vi "Presets.vi"(4 "RLimit":bool, 6 "LLimit":bool, 8 "TwistAxis":dbl, 9 "Key":bool, 10 "STOP":bool, 11 "100":bool) -> ()   [LabVIEW 2011]
uses:
  Manual-Auto.vi
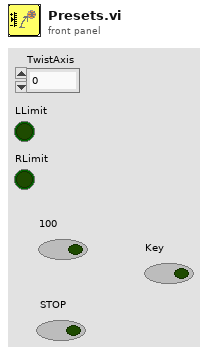
[diagram p1: front panel]
types:
  T1 = typedef "WPI_MotorControlDeviceRef.ctl" = cluster{"DeviceStatus":errorcluster, "Type":enum16{"PWM", "CAN"}, "PWM":cluster{"Digital Module":T2, "PWM Channel":T3, "DeadBand":T4}, "CAN":cluster{"Device Number":u8, "Control Mode":T5, "Semaphore":T6, "Max Vout":dbl}, "Invert":bool, "TransformRef":T7, "InvTransformRef":T7}
  T2 = typedef "FPGA_TypedefDigitalModule.ctl" = enum16{"Digital Module 1", "Digital Module 2"}
  T3 = typedef "FPGA_DIOPWMChannel.ctl" = enum8{"PWM 1", "PWM 2", "PWM 3", "PWM 4", "PWM 5", "PWM 6", "PWM 7", "PWM 8", "PWM 9", "PWM 10", "Invalid"}
  T4 = typedef "WPI_PWMDeadband.ctl" = cluster{"Name":string, "maxPositivePwm":i32, "minPositivePwm":i32, "centerPwm":i32, "maxNegativePwm":i32, "minNegativePwm":i32, "angularRange":u16}
  T5 = typedef "WPI_CANJaguar_ControlMode.ctl" = enum8{"Percent VBus", "Current", "Speed", "Position", "Voltage"}
  T6 = typedef "Semaphore RefNum" = refnum<k1>
  T7 = typedef "WPI_PWMTransform_ConPane.ctl" = refnum<vi>
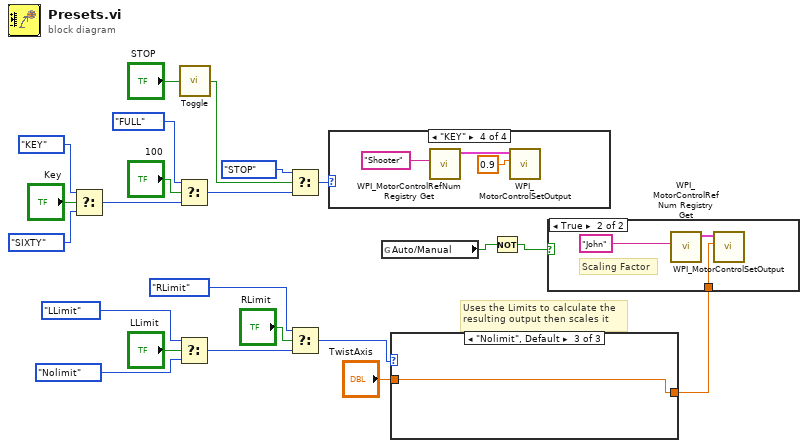
[diagram p0: block diagram]
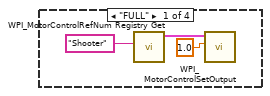
[diagram p3: hidden frame]
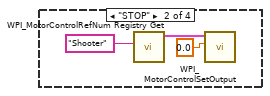
[diagram p4: hidden frame]
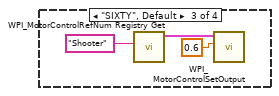
[diagram p5: hidden frame]
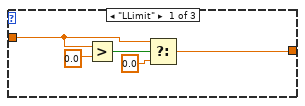
[diagram p6: hidden frame]
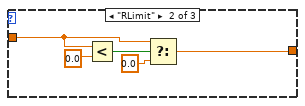
[diagram p7: hidden frame]
diagram:
  # "Uses the Limits to calculate the\nresulting output then scales it"
  n1 = Select(t=enum16{"FULL", "STOP", "SIXTY", "KEY"}."KEY", s="Key", f=enum16{"FULL", "STOP", "SIXTY", "KEY"}."SIXTY") -> (s? t:f=w10:enum16{"FULL", "STOP", "SIXTY", "KEY"})
  n2 = Select(t=enum16{"FULL", "STOP", "SIXTY", "KEY"}."FULL", s="100", f=w10) -> (s? t:f=w13:enum16{"FULL", "STOP", "SIXTY", "KEY"})
  n3 = Select(t=enum16{"LLimit", "RLimit", "Nolimit"}."LLimit", s="LLimit", f=enum16{"LLimit", "RLimit", "Nolimit"}."Nolimit") -> (s? t:f=w20:enum16{"LLimit", "RLimit", "Nolimit"})
  n4 = call "Toggle.vi"("Boolean"="STOP") -> ("Boolean 2"=w3:bool)
  n5 = Select(t=enum16{"FULL", "STOP", "SIXTY", "KEY"}."STOP", s=w3, f=w13) -> (s? t:f=w12:enum16{"FULL", "STOP", "SIXTY", "KEY"})
  n6 = Select(t=enum16{"LLimit", "RLimit", "Nolimit"}."RLimit", s="RLimit", f=w20) -> (s? t:f=w18:enum16{"LLimit", "RLimit", "Nolimit"})
  n7 = case shown="\"KEY\"" w12 {
    frame "FULL" {
      n8 = call <vilib>:"WPI_MotorControlRefNum Registry Get.vi"("refnum name"="Shooter") -> ("MotorControlDevRef"=w23:T1)  [unwired: 9 in, 1 out]
      n9 = call <vilib>:"WPI_MotorControlSetOutput.vi"("Output"=1.0, "MotorControlDevRef"=w23) -> ()  [unwired: 8 in, 2 out]
    }
    frame "STOP" {
      n10 = call <vilib>:"WPI_MotorControlRefNum Registry Get.vi"("refnum name"="Shooter") -> ("MotorControlDevRef"=w28:T1)  [unwired: 9 in, 1 out]
      n11 = call <vilib>:"WPI_MotorControlSetOutput.vi"("Output"=0.0, "MotorControlDevRef"=w28) -> ()  [unwired: 8 in, 2 out]
    }
    frame "SIXTY", Default {
      n12 = call <vilib>:"WPI_MotorControlRefNum Registry Get.vi"("refnum name"="Shooter") -> ("MotorControlDevRef"=w31:T1)  [unwired: 9 in, 1 out]
      n13 = call <vilib>:"WPI_MotorControlSetOutput.vi"("Output"=0.6, "MotorControlDevRef"=w31) -> ()  [unwired: 8 in, 2 out]
    }
    frame "KEY" {
      n14 = call <vilib>:"WPI_MotorControlRefNum Registry Get.vi"("refnum name"="Shooter") -> ("MotorControlDevRef"=w34:T1)  [unwired: 9 in, 1 out]
      n15 = call <vilib>:"WPI_MotorControlSetOutput.vi"("Output"=0.9, "MotorControlDevRef"=w34) -> ()  [unwired: 8 in, 2 out]
    }
  }
  n16 = global read "Manual-Auto.vi" "Auto/Manual"() -> (w2:bool)
  n17 = case shown="\"Nolimit\", Default" w18 {
    tunnel: [w37 w41 w45] -> w17
    tunnel: "TwistAxis" -> [w36 w40 w45]
    frame "LLimit" {
      n18 = Greater?(x=w36, y=0.0) -> (0:w38:bool)
      n19 = Select(t=w36, s=w38, f=0.0) -> (s? t:f=w37:dbl)
    }
    frame "RLimit" {
      n20 = Less?(x=w40, y=0.0) -> (x < y?=w43:bool)
      n21 = Select(t=w40, s=w43, f=0.0) -> (s? t:f=w41:dbl)
    }
    frame "Nolimit", Default {
    }
  }
  n22 = Not(x=w2) -> (.not. x?=w1:bool)
  n23 = case shown="True" w1 {
    tunnel: w17 -> [_ w46]
    frame False {
    }
    frame True {
      # "Scaling Factor"
      n24 = call <vilib>:"WPI_MotorControlRefNum Registry Get.vi"("refnum name"="John") -> ("MotorControlDevRef"=w48:T1)  [unwired: 9 in, 1 out]
      n25 = call <vilib>:"WPI_MotorControlSetOutput.vi"("Output"=w46, "MotorControlDevRef"=w48) -> ()  [unwired: 8 in, 2 out]
    }
  }
